vi "Is Overconsistent.vi"(3 "error in (no error)":errorcluster, 5 "AbstractDstarNode in":refnum<class "NI_Robotics_AbstractDstarNode.lvclass">) -> (0 "error out":errorcluster, 1 "is Overconsistent":bool, 2 "AbstractDstarNode out":refnum<class "NI_Robotics_AbstractDstarNode.lvclass">)   [LabVIEW 2017, in "NI_Robotics_AbstractDstarNode.lvclass"]
uses:
  <vilib>/robotics/Navigation/shared/MapNode/AbstractDstarNode/NI_Robotics_AbstractDstarNode.lvclass
  <vilib>/robotics/Navigation/shared/MapNode/AbstractDstarNode/NI_Robotics_AbstractDstarNode.lvclass/NI_Robotics_AbstractDstarNode.ctl
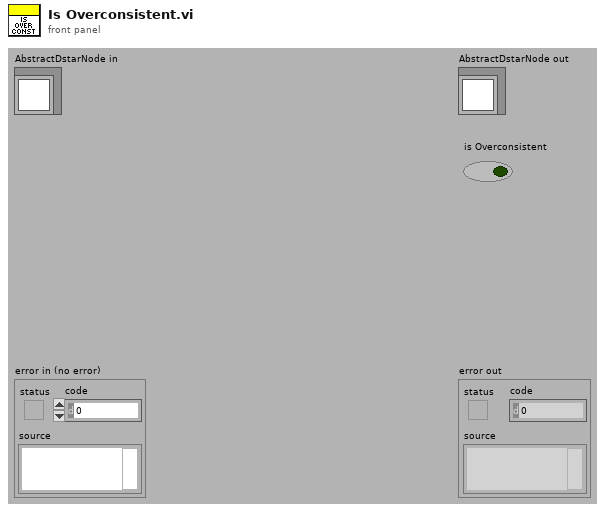
[diagram p1: front panel]
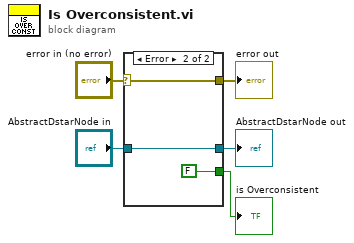
[diagram p0: block diagram]
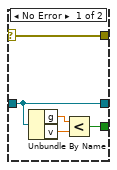
[diagram p2: hidden frame]
diagram:
  n1 = case shown="Error" "error in (no error)" {
    selector: "error in (no error)" -> [w10 w12]
    tunnel: [w10 w12] -> w4
    tunnel: [w6 w13] -> w2
    tunnel: "AbstractDstarNode in" -> [w6 w13]
    tunnel: [w9 FALSE] -> w1
    frame No Error {
      n2 = Unbundle By Name(w6) -> ("g"=w8:dbl, "v"=w7:dbl)
      n3 = Less?(x=w8, y=w7) -> (x < y?=w9:bool)
    }
    frame Error {
    }
  }
  "error out" <- w4
  "AbstractDstarNode out" <- w2
  "is Overconsistent" <- w1
